vi "Kundeneingabe.vi"(8 "error in (no error)":errorcluster) -> (0 "error out":errorcluster)   [LabVIEW 2023]
uses:
  <vilib>/Utility/miscctls.llb/LVRectTypeDef.ctl
panel:
  in  "Front Panel Window:Panel Bounds":T1
  in  "PLZ":dbl
  in  "Ort":string
  in  "Straße":string
  in  "Firmenname":string
  out "Firma":bool
  in  "Blank Button 3":bool
  in  "Blank Button 2":bool
  in  "Blank Button":bool
  in  "Stop Button":bool
  in  "Nachname":string
  in  "Vorname":string
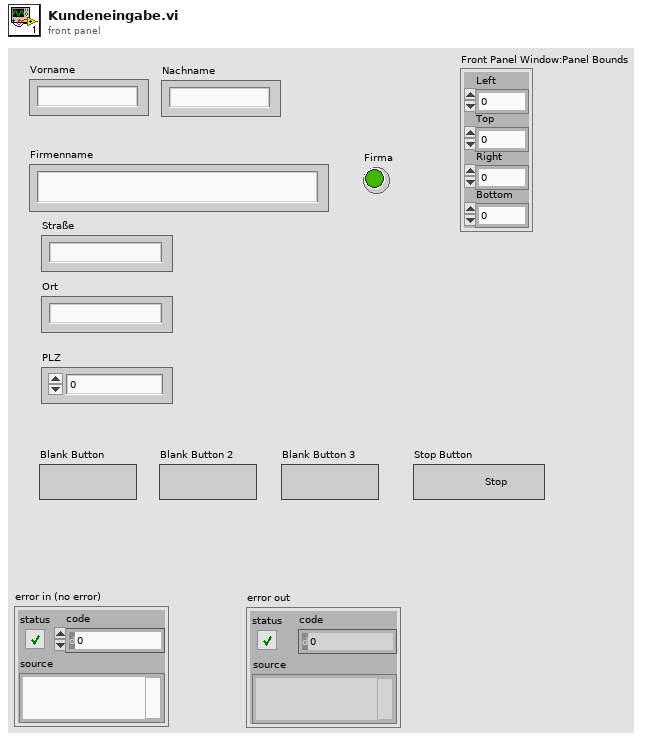
[diagram p1: front panel]
types:
  T1 = typedef "LVRectTypeDef.ctl" = cluster{"Left":i16, "Top":i16, "Right":i16, "Bottom":i16}
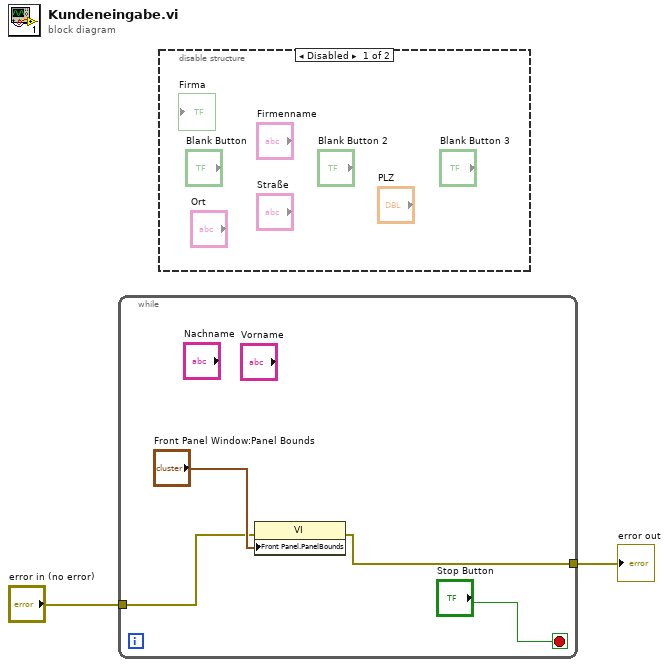
[diagram p0: block diagram]
diagram:
  n1 = while {
    tunnel: "error in (no error)" -> [w4]
    tunnel: [w3] -> w1
    stop <- "Stop Button" stop-if-true
    n2 = property class="VI"(error in=w4, "Front Panel.PanelBounds"="Front Panel Window:Panel Bounds") -> (error out=w3:errorcluster)  [unwired: 1 in, 1 out]
  }
  "error out" <- w1
  n3 = disable-structure shown="Disabled" {
    frame Disabled {
    }
    frame Enabled {
    }
  }
